vi "delete directory contents.vi"(2 "error in":errorcluster, 3 "Directory to delete":path=path "\\\\Enviro\\enviro/Software/RunTime7") -> (0 "error out":errorcluster, 1 "dup directory path":path)   [LabVIEW 2010]
panel:
  out "Current file":string
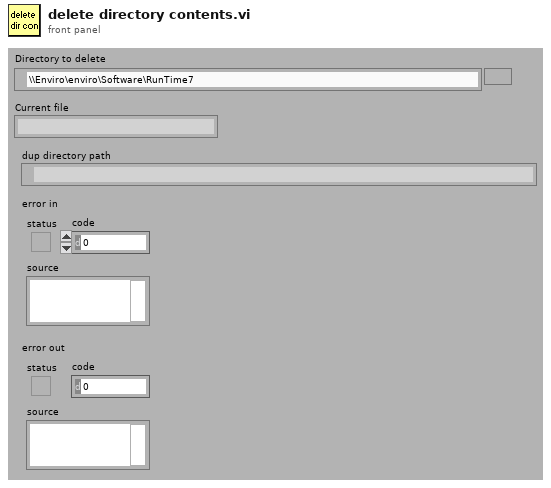
[diagram p1: front panel]
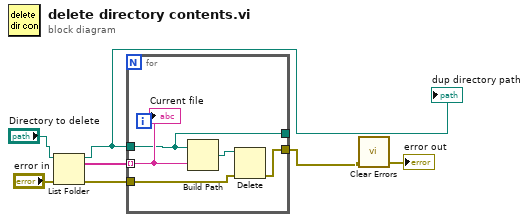
[diagram p0: block diagram]
diagram:
  n1 = List Folder(path="Directory to delete", error in="error in") -> (path out=w2:path, filenames=w6:string[], error out=w5:errorcluster)  [unwired: 2 in, 1 out]
  "dup directory path" <- w2
  n2 = for {
    tunnel: w2 -> [w10]
    tunnel: w6 -> [w11] mode=indexing
    tunnel: [w10] -> _
    tunnel: [w9] -> w1
    tunnel: w5 -> [w8]
    n3 = Build Path(base path=w10, name or relative path=w11) -> (appended path=w12:path)
    n4 = Delete(path (use dialog)=w12, error in=w8) -> (error out=w9:errorcluster)  [unwired: 3 in, 2 out]
    "Current file" <- w11
  }
  n5 = call <vilib>:"Clear Errors.vi"("error in (no error)"=w1) -> ("error out"=→"error out":errorcluster)  [unwired: 6 in]
